vi "Generate Comments.vi"(7 "error in (no error)":errorcluster, 10 "Control Experiment":refnum<class "SMO.Control Experiment.lvclass">) -> (0 "error out":errorcluster, 2 "Comments":string, 3 "Control Experiment out":refnum<class "SMO.Control Experiment.lvclass">)   [LabVIEW 2019, in "SMO.Control Experiment.lvclass"]
uses:
  SMO.Control Experiment.lvclass
  SMO.Control Experiment.lvclass/SMO.Control Experiment.ctl
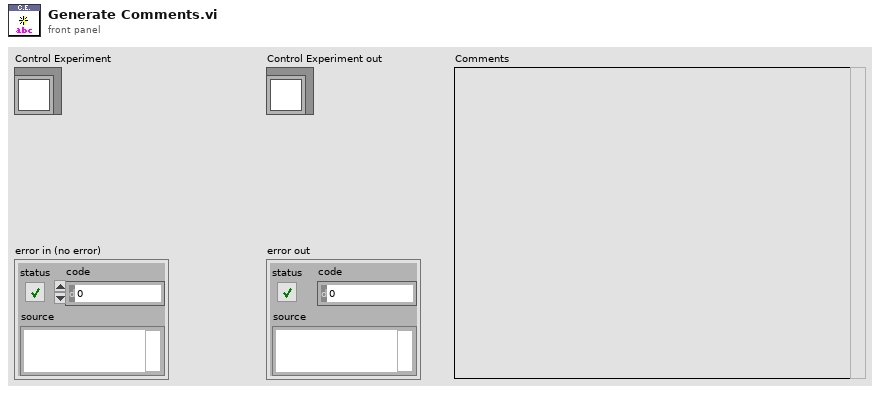
[diagram p1: front panel]
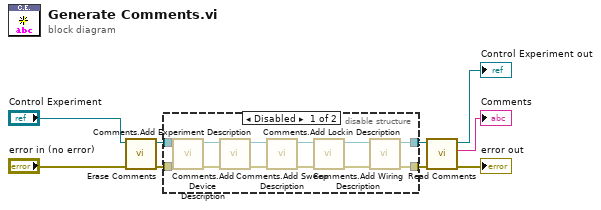
[diagram p0: block diagram]
diagram:
  n1 = call "Erase Comments.vi"("error in (no error)"="error in (no error)", "Control Experiment"="Control Experiment") -> ("error out"=w1:errorcluster, "Control Experiment out"=w3:refnum<class "SMO.Control Experiment.lvclass">)  [unwired: 8 in]
  n2 = disable-structure shown="Disabled" {
    disable-tunnel: [w21 w23] -> w8
    disable-tunnel: [w20 w22] -> w6
    disable-tunnel: w3 -> [w19 w23]
    disable-tunnel: w1 -> [w18 w22]
    frame Disabled {
      n3 = call "Comments.Add Device Description.vi"("error in (no error)"=w18, "Control Experiment"=w19) -> ("error out"=w16:errorcluster, "Control Experiment out"=w17:refnum<class "SMO.Control Experiment.lvclass">)  [unwired: 8 in]
      n4 = call "Comments.Add Experiment Description.vi"("error in (no error)"=w16, "Control Experiment"=w17) -> ("error out"=w12:errorcluster, "Control Experiment out"=w13:refnum<class "SMO.Control Experiment.lvclass">)  [unwired: 7 in]
      n5 = call "Comments.Add Sweep Description.vi"("error in (no error)"=w12, "Control Experiment"=w13) -> ("error out"=w10:errorcluster, "Control Experiment out"=w11:refnum<class "SMO.Control Experiment.lvclass">)  [unwired: 7 in, 1 out]
      n6 = call "Comments.Add Wiring Description.vi"("error in (no error)"=w10, "Control Experiment"=w11) -> ("error out"=w14:errorcluster, "Control Experiment out"=w15:refnum<class "SMO.Control Experiment.lvclass">)  [unwired: 7 in, 1 out]
      n7 = call "Comments.Add Lockin Description.vi"("error in (no error)"=w14, "Control Experiment"=w15) -> ("error out"=w20:errorcluster, "Control Experiment out"=w21:refnum<class "SMO.Control Experiment.lvclass">)  [unwired: 7 in]
    }
    frame Enabled {
    }
  }
  n8 = call "Read Comments.vi"("error in (no error)"=w6, "Control Experiment"=w8) -> ("error out"=→"error out":errorcluster, "Comments"=→"Comments":string, "Control Experiment out"=→"Control Experiment out":refnum<class "SMO.Control Experiment.lvclass">)  [unwired: 7 in]
